vi "Facade.vi"(0 "Data In":T4, 2 "Display State In":T2, 3 "Container State":T3) -> (6 "Data Out":T4, 7 "Display State Out":T2, 8 "Action":T1)   [LabVIEW 2010, in "XControl.xctl"]
uses:
  Xcontrol.xctl
  Data.ctl
  <vilib>/_xctls/Container State.ctl
  State.ctl
  <vilib>/_xctls/Action.ctl
  <vilib>/_xctls/XControlSupport.lvlib
panel:
  out "Graph":cluster{dbl, dbl}[](graph)
  in  "Delete Point":bool
  in  "XY":cluster{"X":dbl, "Y":dbl}
  in  "Add Point":bool
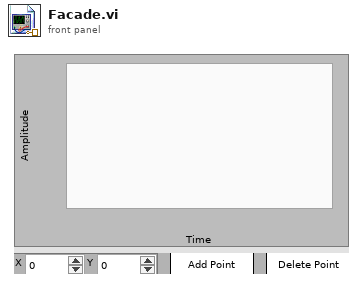
[diagram p1: front panel]
types:
  T1 = typedef "XControlSupport.lvlib/Action.ctl" = cluster{"Data Changed?":bool, "State Changed?":bool, "Action Name":string}
  T2 = typedef "XControl.xctl/State.ctl" = cluster{"Numeric":dbl}
  T3 = typedef "XControlSupport.lvlib/Container State.ctl" = cluster{"Indicator?":bool, "Run Mode?":bool, " Refnum":refnum<vi>}
  T4 = typedef "XControl.xctl/Data.ctl" = cluster{"X":dbl, "Y":dbl}[]
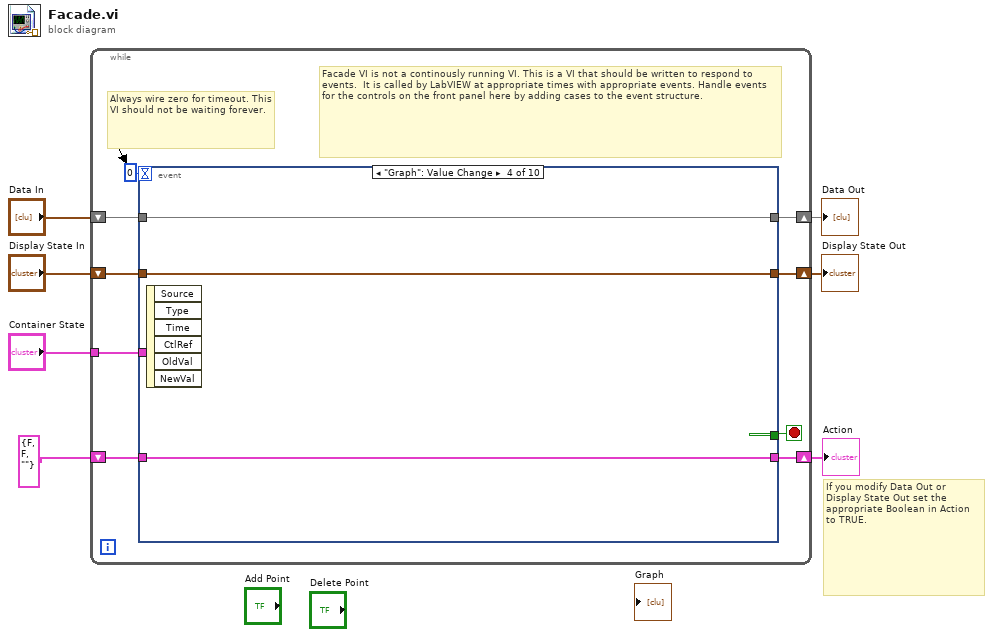
[diagram p0: block diagram]
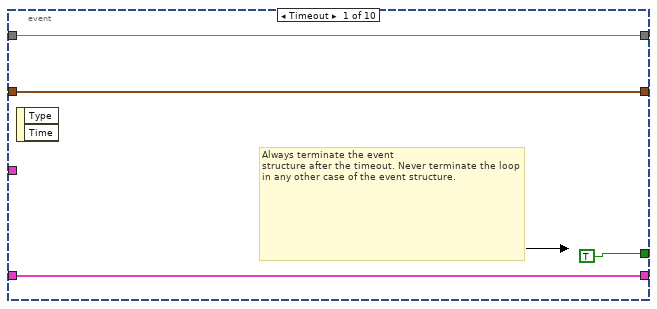
[diagram p2: hidden frame]
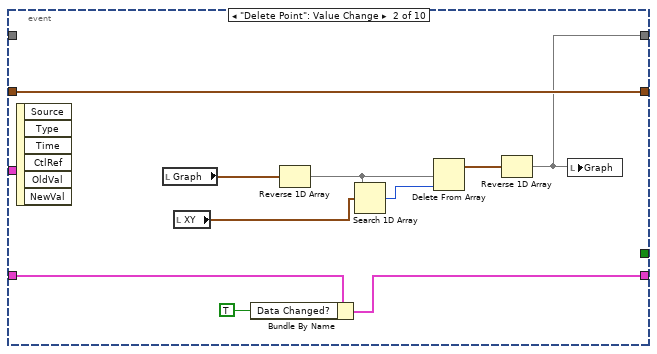
[diagram p3: hidden frame]
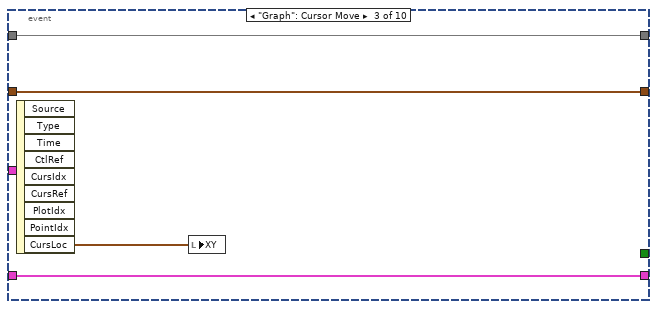
[diagram p4: hidden frame]
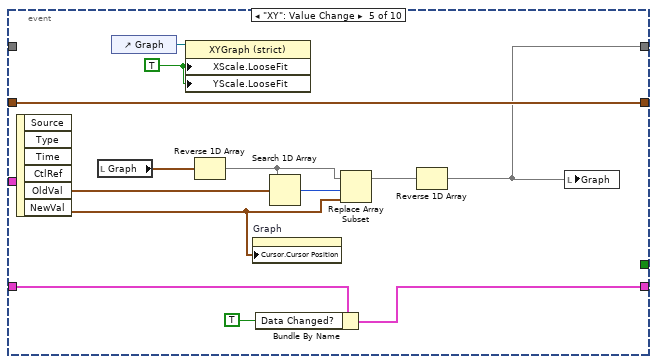
[diagram p5: hidden frame]
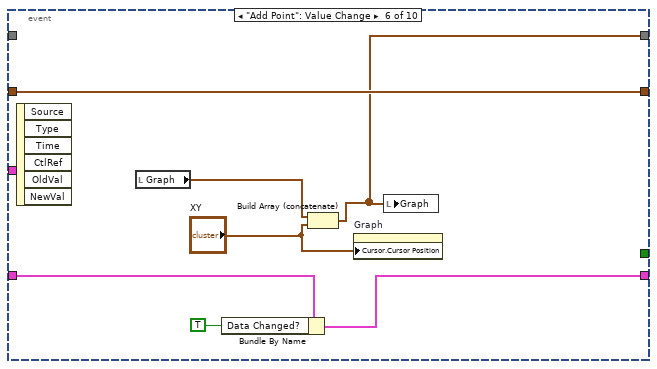
[diagram p6: hidden frame]
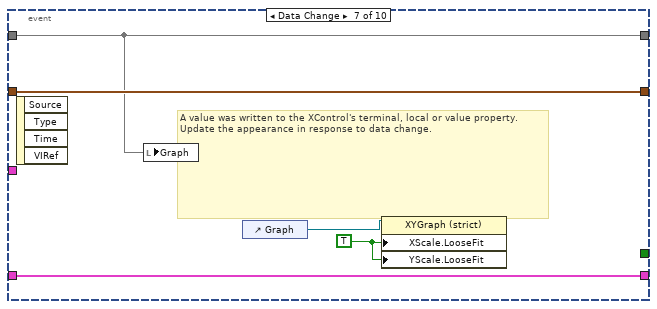
[diagram p7: hidden frame]
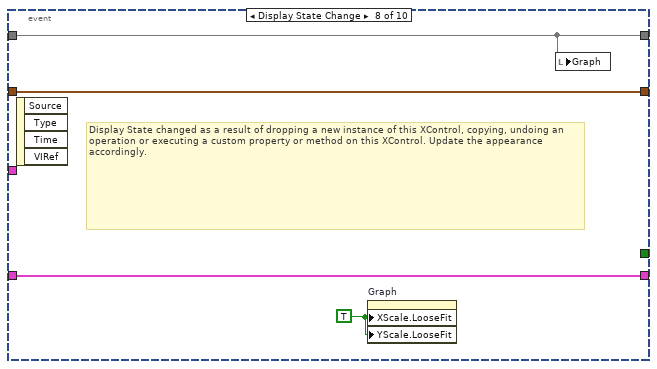
[diagram p8: hidden frame]
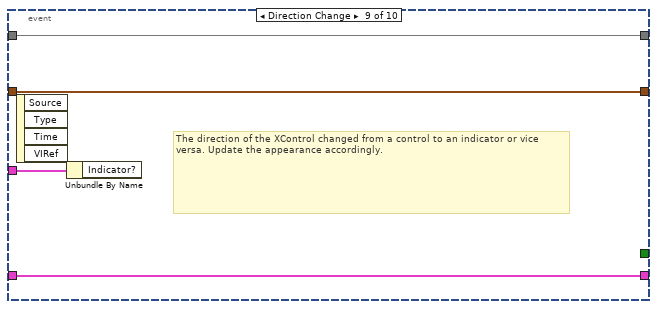
[diagram p9: hidden frame]
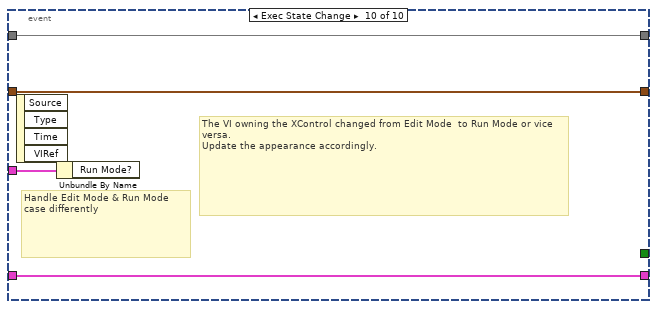
[diagram p10: hidden frame]
diagram:
  # "If you modify Data Out or\nDisplay State Out set the\nappropriate Boolean in Action\nto TRUE."
  n1 = while {
    shift-right: [w15] -> w4
    shift-left: "Display State In" -> [w16]
    tunnel: "Container State" -> [w12]
    shift-right: [w10] -> w7
    shift-left: "Data In" -> [w11]
    shift-right: [w8] -> w2
    shift-left: T1 {"Data Changed?"=FALSE, "State Changed?"=FALSE, "Action Name"=""} ("Action") -> [w9]
    stop <- w14 stop-if-true
    # "Facade VI is not a continously running VI. This is a VI that should be written to respond to events.  It is called by LabVIEW at appropriate times with appropriate events. Handle events for the controls on the front panel here by adding cases to the event structure."
    # "Always wire zero for timeout. This\nVI should not be waiting forever."
    n2 = event shown="[3] \"Graph\": Value Change" {
      selector: _ -> [_ _ _ _ _ _ _ _ _ _]
      dyn-events: _ -> [_ _ _ _ _ _ _ _ _ _]
      timeout: 0 -> [_ _ _ _ _ _ _ _ _ _]
      tunnel: w16 -> [w18 w30 w32 w36 w48 w57 w62 w66 w69 w73]
      tunnel: [w18 w30 w32 w36 w48 w57 w62 w66 w69 w73] -> w15
      tunnel: [TRUE _ _ _ _ _ _ _ _ _] -> w14
      tunnel: w12 -> [_ _ _ _ _ _ _ _ w70 w74]
      tunnel: w11 -> [w17 _ w33 w37 _ _ w60 w64 w68 w72]
      tunnel: [w17 w28 w33 w37 w44 w56 w60 w64 w68 w72] -> w10
      tunnel: [w19 w25 w31 w35 w42 w52 w61 w65 w67 w71] -> w8
      tunnel: w9 -> [w19 w26 w31 w35 w43 w53 w61 w65 w67 w71]
      event Timeout {
        # "Always terminate the event\nstructure after the timeout. Never terminate the loop in any other case of the event structure."
        n3 = event-data() -> ()  [unwired: 1 in, 2 out]
      }
      event "Delete Point": Value Change {
        n4 = event-data() -> ()  [unwired: 1 in, 6 out]
        n5 = local read "Graph"() -> (w29:cluster{dbl, dbl}[])
        n6 = local read "XY"() -> (w21:cluster{"X":dbl, "Y":dbl})
        n7 = Bundle By Name(cluster=w26, "Data Changed?"=TRUE) -> (w25:T1)
        n8 = Reverse 1D Array(array=w29) -> (reversed array=w24:cluster{dbl, dbl}[])
        n9 = Search 1D Array(1D array=w24, element=w21) -> (index of element=w23:i32)  [unwired: 1 in]
        n10 = Delete From Array(array=w24, index=w23) -> (array with subset deleted=w22:cluster{dbl, dbl}[])  [unwired: 1 in, 1 out]
        n11 = Reverse 1D Array(array=w22) -> (reversed array=w28:cluster{dbl, dbl}[])
        n12 = local write "Graph"(w28) -> ()
      }
      event "Graph": Cursor Move {
        n13 = event-data() -> ("CursLoc"=w34:cluster{"X":dbl, "Y":dbl})  [unwired: 1 in, 8 out]
        n14 = local write "XY"(w34) -> ()
      }
      event "Graph": Value Change {
        n15 = event-data() -> ()  [unwired: 1 in, 6 out]
      }
      event "XY": Value Change {
        w40 = TRUE ("X Scale.Loose Fit")
        n16 = event-data() -> ("OldVal"=w49:cluster{"X":dbl, "Y":dbl}, "NewVal"=w38:cluster{"X":dbl, "Y":dbl})  [unwired: 1 in, 4 out]
        n17 = local read "Graph"() -> (w47:cluster{dbl, dbl}[])
        n18 = control-ref of="Graph"() -> (w39:refnum<vi>)
        n19 = property on="Property Node" class="XYGraph (strict)"(reference=w39, "XScale.LooseFit"=w40, "YScale.LooseFit"=w40) -> ()  [unwired: 1 in, 2 out]
        n20 = Reverse 1D Array(array=w47) -> (reversed array=w46:cluster{dbl, dbl}[])
        n21 = property on="Graph" class="XYGraph (strict)"("Cursor.Cursor Position"=w38) -> ()  [unwired: 2 in, 2 out]
        n22 = Bundle By Name(cluster=w43, "Data Changed?"=TRUE) -> (w42:T1)
        n23 = Search 1D Array(1D array=w46, element=w49) -> (index of element=w50:i32)  [unwired: 1 in]
        n24 = Replace Array Subset(array=w46, new element=w38, index=w50) -> (w45:cluster{dbl, dbl}[])
        n25 = Reverse 1D Array(array=w45) -> (reversed array=w44:cluster{dbl, dbl}[])
        n26 = local write "Graph"(w44) -> ()
      }
      event "Add Point": Value Change {
        n27 = event-data() -> ()  [unwired: 1 in, 6 out]
        n28 = local read "Graph"() -> (w55:cluster{dbl, dbl}[])
        n29 = Bundle By Name(cluster=w53, "Data Changed?"=TRUE) -> (w52:T1)
        n30 = Build Array (concatenate)(w55, "XY") -> (w56:cluster{"X":dbl, "Y":dbl}[])
        n31 = property on="Graph" class="XYGraph (strict)"("Cursor.Cursor Position"="XY") -> ()  [unwired: 2 in, 2 out]
        n32 = local write "Graph"(w56) -> ()
      }
      event Data Change {
        w59 = TRUE ("X Scale.Loose Fit")
        # "A value was written to the XControl's terminal, local or value property.\nUpdate the appearance in response to data change."
        n33 = event-data() -> ()  [unwired: 1 in, 4 out]
        n34 = local write "Graph"(w60) -> ()
        n35 = control-ref of="Graph"() -> (w58:refnum<vi>)
        n36 = property on="Property Node" class="XYGraph (strict)"(reference=w58, "XScale.LooseFit"=w59, "YScale.LooseFit"=w59) -> ()  [unwired: 1 in, 2 out]
      }
      event Display State Change {
        w63 = TRUE ("X Scale.Loose Fit")
        # "Display State changed as a result of dropping a new instance of this XControl, copying, undoing an operation or executing a custom property or method on this XControl. Update the appearance accordingly."
        n37 = event-data() -> ()  [unwired: 1 in, 4 out]
        n38 = property on="Graph" class="XYGraph (strict)"("XScale.LooseFit"=w63, "YScale.LooseFit"=w63) -> ()  [unwired: 2 in, 2 out]
        n39 = local write "Graph"(w64) -> ()
      }
      event Direction Change {
        # "The direction of the XControl changed from a control to an indicator or vice versa. Update the appearance accordingly."
        n40 = event-data() -> ()  [unwired: 1 in, 4 out]
        n41 = Unbundle By Name(w70) -> ()  [unwired: 1 out]
      }
      event Exec State Change {
        # "The VI owning the XControl changed from Edit Mode  to Run Mode or vice versa.\nUpdate the appearance accordingly."
        # "Handle Edit Mode & Run Mode\ncase differently"
        n42 = event-data() -> ()  [unwired: 1 in, 4 out]
        n43 = Unbundle By Name(w74) -> ()  [unwired: 1 out]
      }
    }
  }
  "Display State Out" <- w4
  "Data Out" <- w7
  "Action" <- w2
